vi "__34401A_init.vi"(7 "GPIB":string="22") -> (0 "error out":errorcluster caption="エラー出力")   [LabVIEW 2017]
panel:
  in  "voltrange(mV)":dbl=10.0
  in  "PLC":dbl=1.0
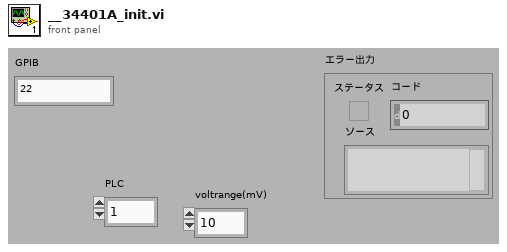
[diagram p1: front panel]
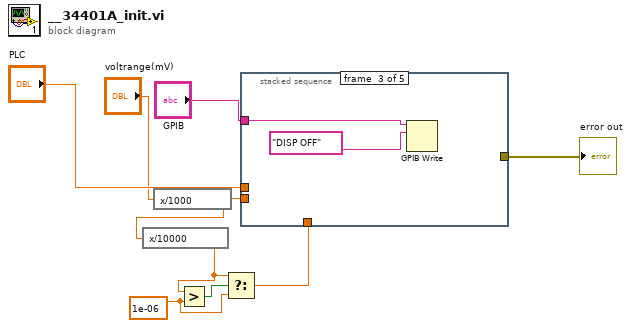
[diagram p0: block diagram]
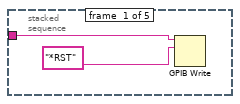
[diagram p2: hidden frame]
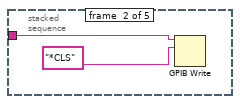
[diagram p3: hidden frame]
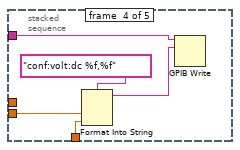
[diagram p4: hidden frame]
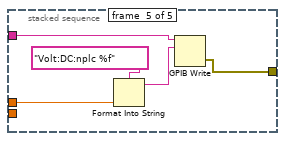
[diagram p5: hidden frame]
diagram:
  w3 = 1e-06
  n1 = expression code="x/1000"("voltrange(mV)") -> (w6:dbl)
  n2 = expression code="x/10000"(w6) -> (w4:dbl)
  n3 = Greater?(x=w4, y=w3) -> (0:w5:bool)
  n4 = Select(t=w4, s=w5, f=w3) -> (s? t:f=w2:dbl)
  n5 = stacked-sequence {
    tunnel: "GPIB" -> [w11 w13 w15 w20 w25]
    tunnel: "PLC" -> [_ _ _ _ w23]
    tunnel: w6 -> [_ _ _ w17 _]
    tunnel: w2 -> [_ _ _ w16 _]
    tunnel: [_ _ _ _ w21] -> w1
    frame #0 {
      n6 = GPIB Write(0:w11, 1:"*RST") -> ()  [unwired: 3 in, 2 out]
    }
    frame #1 {
      n7 = GPIB Write(0:w13, 1:"*CLS") -> ()  [unwired: 3 in, 2 out]
    }
    frame #2 {
      n8 = GPIB Write(0:w15, 1:"DISP OFF") -> ()  [unwired: 3 in, 2 out]
    }
    frame #3 {
      n9 = Format Into String(format string="conf:volt:dc %f,%f", w17, w16) -> (resulting string=w18:string)  [unwired: 2 in, 1 out]
      n10 = GPIB Write(0:w20, 1:w18) -> ()  [unwired: 3 in, 2 out]
    }
    frame #4 {
      n11 = Format Into String(format string="Volt:DC:nplc %f", w23) -> (resulting string=w22:string)  [unwired: 2 in, 1 out]
      n12 = GPIB Write(0:w25, 1:w22) -> (6:w21:errorcluster)  [unwired: 3 in, 1 out]
    }
  }
  "error out" <- w1
